vi "configure piezo and pockelscontrol for galvo.vi"() -> (0 "error out":errorcluster, 3 "Array of Piezo and Pockels Task":refnum<k21>[](array[refnum]))   [LabVIEW 2017]
doc: "SciScan 1.2 160622"
uses:
  <vilib>/DAQmx/write.llb/DAQmx Write (Analog 2D DBL NChan NSamp).vi
  <vilib>/DAQmx/write.llb/DAQmx Write (Analog 1D DBL 1Chan NSamp).vi
  GFG/GFGstringGet.vi
  GFG/GFGfpRefGet.vi
  GFG/GFGnumericGet.vi
  GFG/GFGbooleanGet.vi
  <vilib>/DAQmx/create/channels.llb/DAQmx Create Channel (AO-Voltage-Basic).vi
  <vilib>/DAQmx/miscellaneous.llb/DAQmx Fill In Error Info.vi
  <vilib>/DAQmx/configure/trigger.llb/DAQmx Start Trigger (Digital Edge).vi
  GFG/GFG library.lvlib
  <resource>/objmgr/daqmx.rc
panel:
  out "error out 2":errorcluster
  out "pockels cell control":dbl[](graph)
  out "piezo control":dbl[](graph)
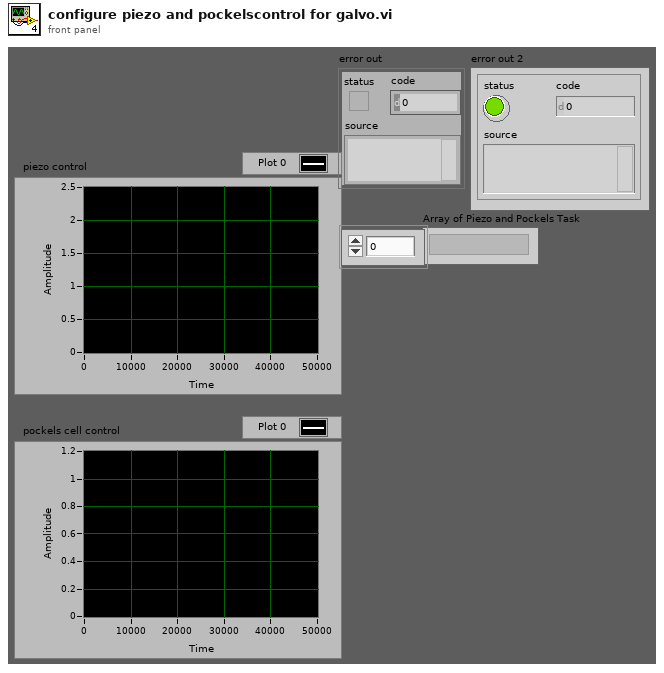
[diagram p1: front panel]
types:
  T1 = enum8{"Enabled", "Disabled", "Disabled and Grayed Out"}
  T2 = cluster{"WaveformChartRef":refnum<vi>, "DigitalRef":refnum<vi>, "ArrayRef":refnum<vi>, "TabControlRef":refnum<vi>, "EnumRef":refnum<vi>, "RingRef":refnum<vi>, "BooleanRef":refnum<vi>, "KnobRef":refnum<vi>, "SlideRef":refnum<vi>, "PathRef":refnum<vi>, "StringRef":refnum<vi>, "ComboBox":refnum<vi>, "WaveformGraphRef":refnum<vi>}
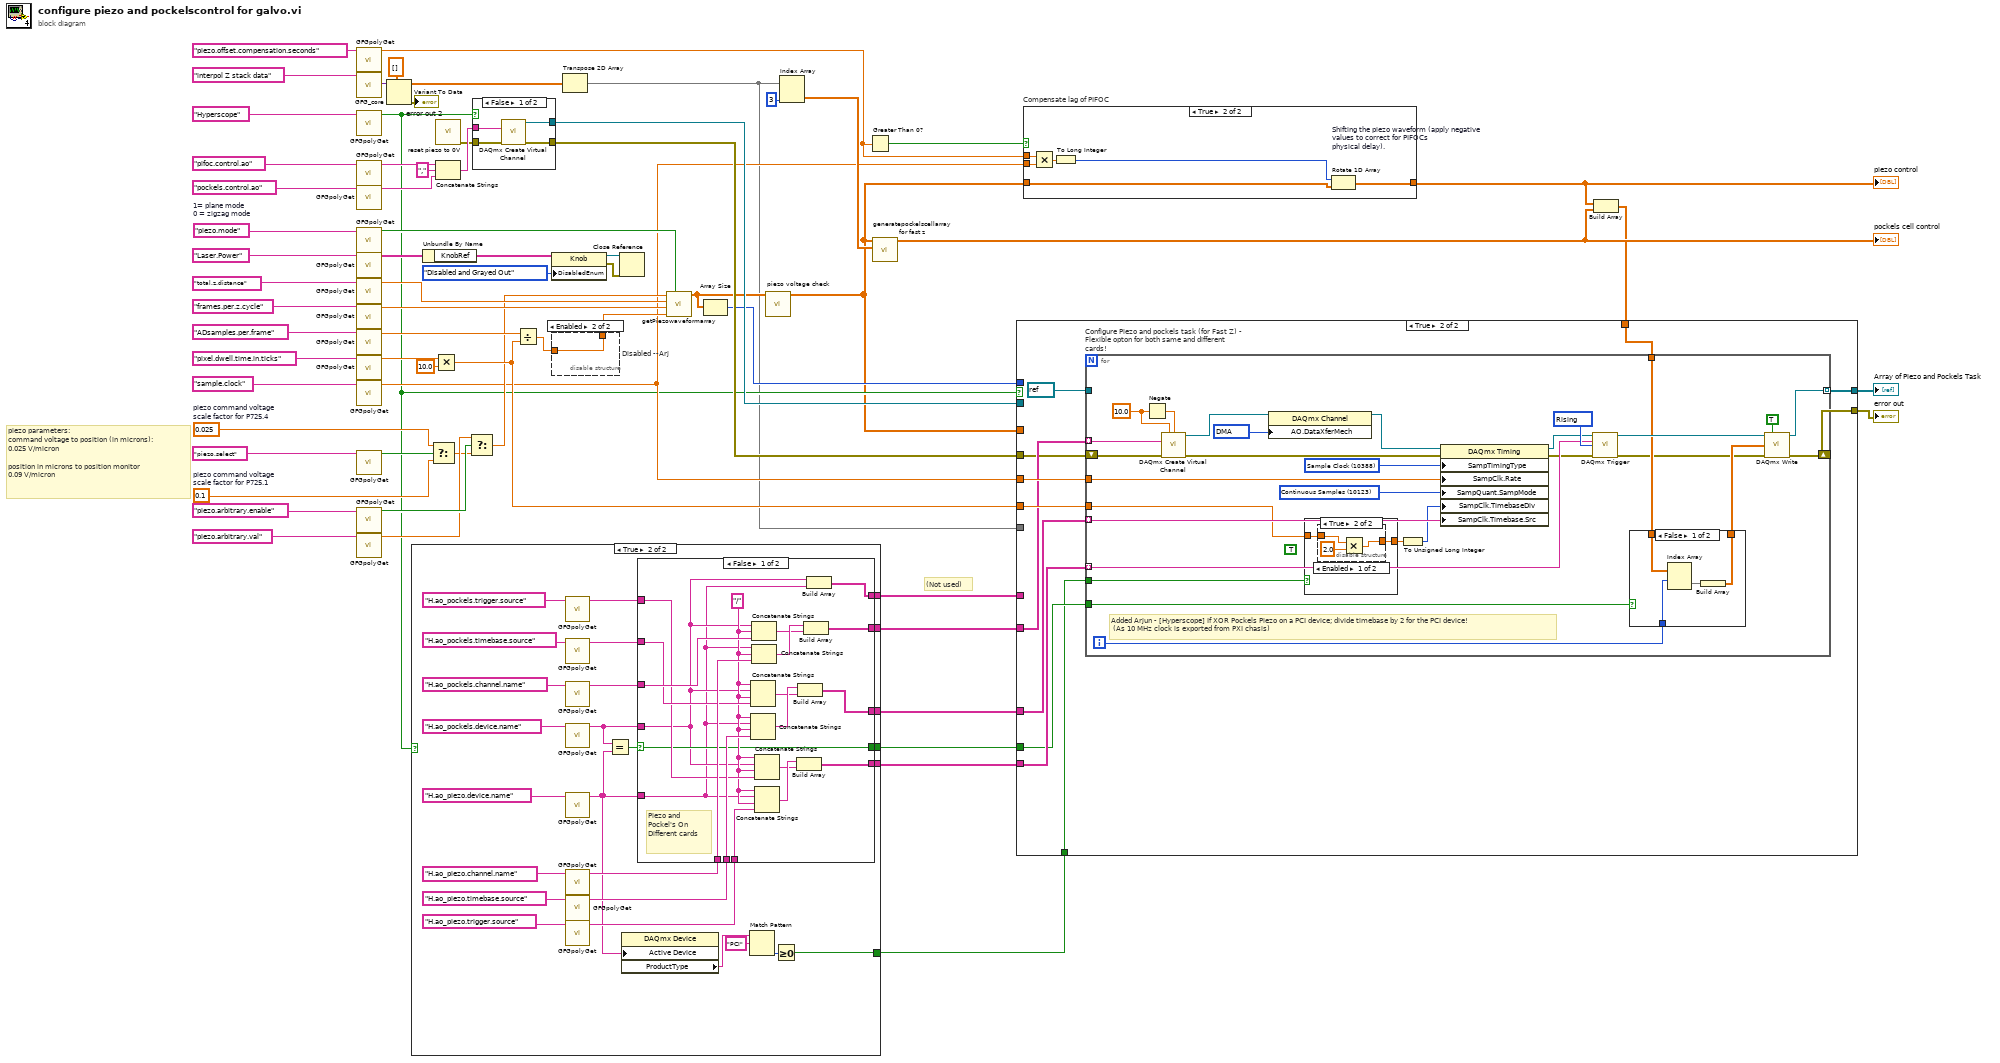
[diagram p0: block diagram]
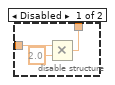
[diagram p2: hidden frame]
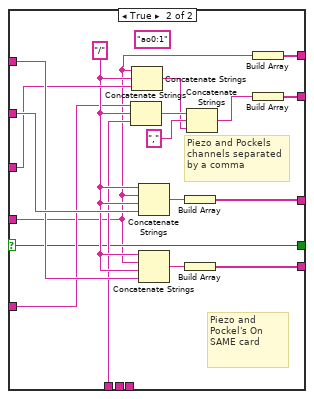
[diagram p4: hidden frame]
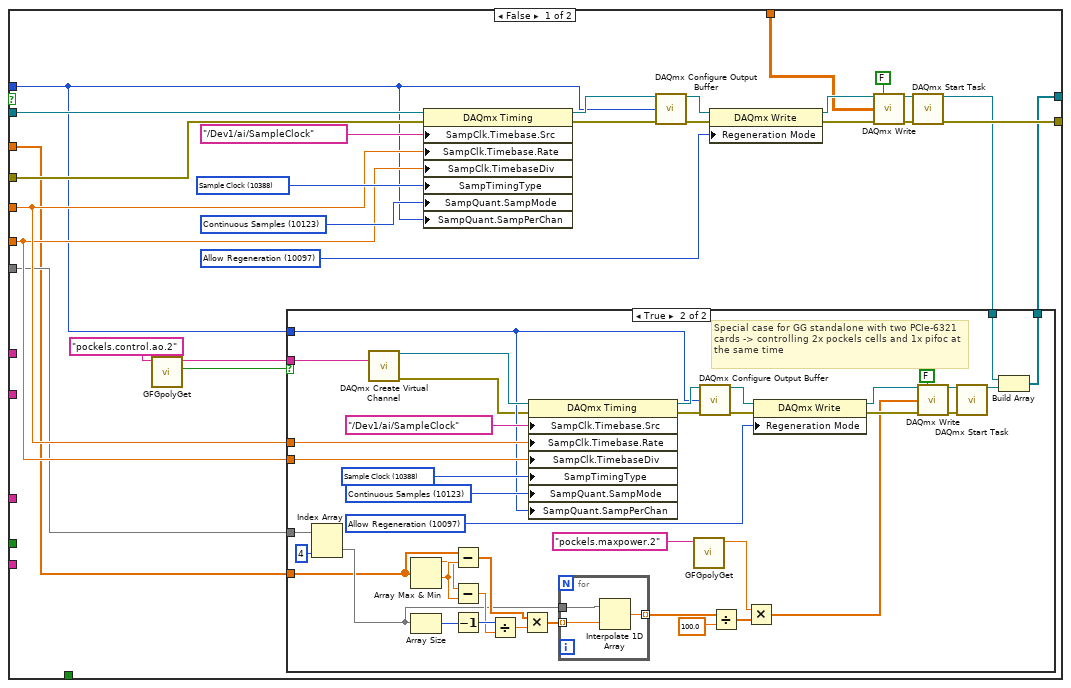
[diagram p6: hidden frame]
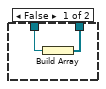
[diagram p7: hidden frame]
diagram:
  w37 = 0.1  # piezo command voltage scale factor for P725.1
  w38 = 0.025  # piezo command voltage scale factor for P725.4
  w48 = "piezo.mode"  # 1= plane mode 0 = zigzag mode
  # "(Not used)"
  # "piezo parameters:\ncommand voltage to position (in microns):\n0.025 V/micron\n\nposition in microns to position monitor\n0.09 V/micron"
  n1 = call-poly "GFGpolyGet.vi"("Variable Name in"="piezo.offset.compensation.seconds") -> ("Numeric"=w16:dbl)  [unwired: 8 in, 2 out]
  n2 = call "GFG_core.vi"("Variable Name in"="interpol Z stack data") -> ("Variant Out"=w47:variant)  [unwired: 12 in, 6 out]
  n3 = call-poly "GFGpolyGet.vi"("Variable Name in"="Hyperscope") -> ("Boolean Value OUT"=w5:bool)  [unwired: 9 in, 1 out]
  n4 = call-poly "GFGpolyGet.vi"("Variable Name in"="pifoc.control.ao") -> ("String"=w65:string)  [unwired: 9 in, 1 out]
  n5 = call-poly "GFGpolyGet.vi"("Variable Name in"="pockels.control.ao" ("Tag in")) -> ("String"=w64:string)  [unwired: 9 in, 1 out]
  n6 = call-poly "GFGpolyGet.vi"("Variable Name in"=w48) -> ("Boolean Value OUT"=w43:bool)  [unwired: 9 in, 1 out]
  n7 = call-poly "GFGpolyGet.vi"("Variable Name in"="Laser.Power") -> ("output cluster"=w62:T2)  [unwired: 9 in, 1 out]
  n8 = call-poly "GFGpolyGet.vi"("Variable Name in"="total.z.distance") -> ("Numeric"=w32:dbl)  [unwired: 8 in, 2 out]
  n9 = call-poly "GFGpolyGet.vi"("Variable Name in"="frames.per.z.cycle" ("Tag in")) -> ("Numeric"=w49:dbl)  [unwired: 8 in, 2 out]
  n10 = call-poly "GFGpolyGet.vi"("Variable Name in"="ADsamples.per.frame" ("Tag in")) -> ("Numeric"=w51:dbl)  [unwired: 8 in, 2 out]
  n11 = call-poly "GFGpolyGet.vi"("Variable Name in"="pixel.dwell.time.in.ticks" ("Tag in")) -> ("Numeric"=w53:dbl)  [unwired: 8 in, 2 out]
  n12 = call-poly "GFGpolyGet.vi"("Variable Name in"="sample.clock" ("Tag in")) -> ("Numeric"=w14:dbl)  [unwired: 8 in, 2 out]
  n13 = call-poly "GFGpolyGet.vi"("Variable Name in"="piezo.select") -> ("Boolean Value OUT"=w35:bool)  [unwired: 9 in, 1 out]
  n14 = call-poly "GFGpolyGet.vi"("Variable Name in"="piezo.arbitrary.enable") -> ("Boolean Value OUT"=w27:bool)  [unwired: 9 in, 1 out]
  n15 = call-poly "GFGpolyGet.vi"("Variable Name in"="piezo.arbitrary.val" ("Tag in")) -> ("Numeric"=w26:dbl)  [unwired: 8 in, 2 out]
  n16 = Variant To Data(type=dbl[][] [] ("Interpolated Data"), Variant=w47) -> (data=w45:dbl[][], error out=→"error out 2":errorcluster)  [unwired: 1 in]
  n17 = case shown="True" w5 {
    tunnel: [_ w79] -> w21
    tunnel: [_ w78] -> w20
    tunnel: [_ w77] -> w19
    tunnel: [_ w75] -> w6
    tunnel: [_ w74] -> w2
    tunnel: [_ w69] -> w1
    frame False {
    }
    frame True {
      n18 = call-poly "GFGpolyGet.vi"("Variable Name in"="H.ao_pockels.trigger.source" ("Tag in")) -> ("String"=w80:string)  [unwired: 9 in, 1 out]
      n19 = call-poly "GFGpolyGet.vi"("Variable Name in"="H.ao_pockels.timebase.source" ("Tag in")) -> ("String"=w81:string)  [unwired: 9 in, 1 out]
      n20 = call-poly "GFGpolyGet.vi"("Variable Name in"="H.ao_pockels.channel.name" ("Tag in")) -> ("String"=w82:string)  [unwired: 9 in, 1 out]
      n21 = call-poly "GFGpolyGet.vi"("Variable Name in"="H.ao_pockels.device.name" ("Tag in")) -> ("String"=w92:string)  [unwired: 9 in, 1 out]
      n22 = call-poly "GFGpolyGet.vi"("Variable Name in"="H.ao_piezo.device.name" ("Tag in")) -> ("String"=w70:string)  [unwired: 9 in, 1 out]
      n23 = call-poly "GFGpolyGet.vi"("Variable Name in"="H.ao_piezo.channel.name" ("Tag in")) -> ("String"=w85:string)  [unwired: 9 in, 1 out]
      n24 = call-poly "GFGpolyGet.vi"("Variable Name in"="H.ao_piezo.timebase.source" ("Tag in")) -> ("String"=w84:string)  [unwired: 9 in, 1 out]
      n25 = call-poly "GFGpolyGet.vi"("Variable Name in"="H.ao_piezo.trigger.source" ("Tag in")) -> ("String"=w83:string)  [unwired: 9 in, 1 out]
      n26 = Equal?(x=w92, y=w70) -> (x = y?=w76:bool)
      n27 = property class="DAQmx Device"("Active Device"=w70) -> ("ProductType"=w73:string)  [unwired: 2 in, 2 out]
      n28 = case shown="False" w76 {
        selector: w76 -> [w98 w117]
        tunnel: w92 -> [w97 w116]
        tunnel: w85 -> [w113 w123]
        tunnel: w84 -> [w110 _]
        tunnel: w83 -> [w107 _]
        tunnel: w70 -> [w96 w122]
        tunnel: w82 -> [w114 w125]
        tunnel: w81 -> [w111 w131]
        tunnel: w80 -> [w109 w126]
        tunnel: [w112 w132] -> w79
        tunnel: [w105 w129] -> w78
        tunnel: [w106 w127] -> w77
        tunnel: [w98 w117] -> w75
        tunnel: [w95 w115] -> w74
        frame False {
          w108 = "/" ("Tag in")
          # "Piezo and Pockel's On Different cards"
          n29 = Concatenate Strings(w108, w97, w108, w111) -> (w101:string)
          n30 = Concatenate Strings(w108, w96, w108, w110) -> (w102:string)
          n31 = Concatenate Strings(w97, w108, w114) -> (w103:string)
          n32 = Concatenate Strings(w96, w108, w113) -> (w104:string)
          n33 = Concatenate Strings(w108, w97, w108, w109) -> (w99:string)
          n34 = Concatenate Strings(w108, w96, w108, w107) -> (w100:string)
          n35 = Build Array(w100, w99) -> (w106:string[])
          n36 = Build Array(w102, w101) -> (w105:string[])
          n37 = Build Array(w104, w103) -> (w112:string[])
          n38 = Build Array(w97, w96) -> (w95:string[])
        }
        frame True {
          (unwired) "ao0:1" ("string")
          w124 = "/" ("Tag in")
          # "Piezo and Pockels channels separated by a comma"
          # "Piezo and Pockel's On SAME card"
          n39 = Concatenate Strings(w122, w124, w123) -> (w121:string)
          n40 = Concatenate Strings(w116, w124, w125) -> (w119:string)
          n41 = Concatenate Strings(w124, w116, w124, w131) -> (w130:string)
          n42 = Concatenate Strings(w124, w116, w124, w126) -> (w128:string)
          n43 = Build Array(w130) -> (w129:string[])
          n44 = Build Array(w128) -> (w127:string[])
          n45 = Concatenate Strings(w121, "," ("string"), w119) -> (w118:string)
          n46 = Build Array(w116) -> (w115:string[])
          n47 = Build Array(w118) -> (w132:string[])
        }
      }
      n48 = Match Pattern(string=w73, regular expression="PCI") -> (offset past match=w71:i32)  [unwired: 1 in, 3 out]
      n49 = Greater Or Equal To 0?(x=w71) -> (x >= 0?=w69:bool)
    }
  }
  n50 = Unbundle By Name(w62) -> ("KnobRef"=w61:refnum<vi>)
  n51 = Select(t=w38, s=w35, f=w37) -> (s? t:f=w25:dbl)
  n52 = Multiply(x=w53, y=10.0) -> (x*y=w31:dbl)
  n53 = call "reset piezo to 0V.vi"() -> ("error out"=w40:errorcluster)  [unwired: 11 in]
  n54 = Concatenate Strings(w65, "," ("string"), w64) -> (w55:string)
  n55 = Select(t=w26, s=w27, f=w25) -> (s? t:f=w24:dbl)
  n56 = case shown="False" w5 {
    tunnel: [w136 w137] -> w59
    tunnel: [w135 _] -> w58
    tunnel: w55 -> [w134 _]
    tunnel: w40 -> [w133 w137]
    frame False {
      n57 = call-poly <vilib>:"DAQmx Create Virtual Channel.vi"("physical channels"=w134, "error in"=w133) -> ("task out"=w135:refnum<k21>, "error out"=w136:errorcluster)  [unwired: 12 in]
    }
    frame True {
    }
  }
  n58 = Divide(x=w51, y=w31) -> (x/y=w7:dbl)
  n59 = property class="Knob"(reference=w61, "DisabledEnum"=T1."Disabled and Grayed Out" ("Disabled")) -> (reference out=w9:refnum<vi>, error out=w8:errorcluster)  [unwired: 1 in]
  n60 = disable-structure "Disabled --Arj" shown="Enabled" {
    disable-tunnel: [w140 w141] -> w57
    disable-tunnel: w7 -> [w139 w141]
    frame Disabled {
      n61 = Multiply(x=w139, y=2.0) -> (x*y=w140:dbl)
    }
    frame Enabled {
    }
  }
  n62 = Transpose 2D Array(2D array=w45) -> (transposed array=w4:dbl[][])
  n63 = Close Reference(reference=w9, error in (no error)=w8) -> ()  [unwired: 1 out]
  n64 = call "getPiezowaveformarray.vi"("sawtooth or zigzag"=w43, "pixel.num"=w57, "frames.per.z.cycle"=w49, "total.z.distance"=w32, "piezo scale factor"=w24) -> ("Array"=w13:dbl[])  [unwired: 6 in]
  n65 = Array Size(array=w13) -> (size(s)=w56:i32)
  n66 = call "piezo voltage check.vi"("piezo array in"=w13) -> ("piezo array out"=w3:dbl[])  [unwired: 10 in]
  n67 = Index Array(array=w4, index (col)=3 ("disabled index (col)")) -> (element=w42:dbl[])  [unwired: 1 in]
  n68 = Greater Than 0?(x=w16) -> (x > 0?=w15:bool)
  n69 = call "generatepockelscellarray for fast z.vi"("interpolated pockels cell data"=w42, "piezo control"=w3) -> ("pockelscellarray"=w11:dbl[])  [unwired: 9 in]
  "pockels cell control" <- w11
  n70 = case "Compensate lag of PIFOC" shown="True" w15 {
    tunnel: w3 -> [w142 w145]
    tunnel: [w142 w143] -> w12
    tunnel: w16 -> [_ w148]
    tunnel: w14 -> [_ w146]
    frame False {
    }
    frame True {
      n71 = Multiply(x=w148, y=w146) -> (x*y=w147:dbl)
      n72 = To Long Integer(number=w147) -> (32bit integer=w144:i32)
      n73 = Rotate 1D Array "Shifting the piezo waveform (apply negative values to correct for PIFOCs\nphysical delay)."(1:w145, 2:w144) -> (0:w143:dbl[])
    }
  }
  "piezo control" <- w12
  n74 = Build Array(w12, w11) -> (w10:dbl[][])
  n75 = case shown="True" w5 {
    tunnel: w59 -> [w169 w224]
    tunnel: w58 -> [w167 _]
    tunnel: w56 -> [w151 _]
    tunnel: w10 -> [w156 w232]
    tunnel: w14 -> [w153 w230]
    tunnel: [w154 w231] -> w18
    tunnel: [w160 w223] -> w39
    tunnel: w31 -> [w152 w229]
    tunnel: w21 -> [_ w226]
    tunnel: w20 -> [_ w227]
    tunnel: w19 -> [_ w228]
    tunnel: w6 -> [_ w225]
    tunnel: w4 -> [w150 _]
    tunnel: w3 -> [w149 _]
    tunnel: w2 -> [_ _]
    tunnel: w1 -> [_ w221]
    frame False {
      w166 = 10388 items=["Sample Clock"=10388, "Burst Handshake"=12548, "Handshake"=10389, "Implicit"=10451, "On Demand"=10390, "Change Detection"=12504, "Pipelined Sample Clock"=14668] ("SampTimingType")
      w174 = 10097 items=["Allow Regeneration"=10097, "Do Not Allow Regeneration"=10158] ("RegenMode")
      w165 = 10123 items=["Finite Samples"=10178, "Continuous Samples"=10123] ("sample mode")
      n76 = call-poly "GFGpolyGet.vi"("Variable Name in"="pockels.control.ao.2" ("Tag in")) -> ("Found/Replaced"=w158:bool, "String"=w157:string)  [unwired: 9 in]
      n77 = property class="DAQmx Timing"(reference=w167, error in=w169, "SampClk.Timebase.Src"=tag "/Dev1/ai/SampleClock" ("Clock Source"), "SampClk.Timebase.Rate"=w153, "SampClk.TimebaseDiv"=w152, "SampTimingType"=w166, "SampQuant.SampMode"=w165, "SampQuant.SampPerChan"=w151) -> (reference out=w163:refnum<k21>, error out=w170:errorcluster)
      n78 = call <vilib>:"DAQmx Configure Output Buffer.vi"("task/channels in"=w163, "buffer size (in samples per channel)"=w151, "error in"=w170) -> ("task out"=w175:refnum<k21>, "error out"=w173:errorcluster)  [unwired: 11 in]
      n79 = property class="DAQmx Write"(reference=w175, error in=w173, "Regeneration Mode"=w174) -> (reference out=w171:refnum<k21>, error out=w172:errorcluster)
      n80 = call-poly <vilib>:"DAQmx Write.vi"("task/channels in"=w171, "auto start"=FALSE, "data"=w156, "error in"=w172) -> ("task out"=w162:refnum<k21>, "error out"=w164:errorcluster)  [unwired: 9 in, 1 out]
      n81 = call <vilib>:"DAQmx Start Task.vi"("task/channels in"=w162, "error in"=w164) -> ("task out"=w155:refnum<k21>, "error out"=w160:errorcluster)  [unwired: 12 in]
      n82 = case shown="True" w158 {
        tunnel: w157 -> [_ w217]
        tunnel: w155 -> [w177 w202]
        tunnel: [w176 w200] -> w154
        tunnel: w153 -> [_ w199]
        tunnel: w152 -> [_ w198]
        tunnel: w151 -> [_ w197]
        tunnel: w150 -> [_ w194]
        tunnel: w149 -> [_ w178]
        frame False {
          n83 = Build Array(w177) -> (w176:refnum<k21>[])
        }
        frame True {
          w211 = 10388 items=["Sample Clock"=10388, "Burst Handshake"=12548, "Handshake"=10389, "Implicit"=10451, "On Demand"=10390, "Change Detection"=12504, "Pipelined Sample Clock"=14668] ("SampTimingType")
          w205 = 10097 items=["Allow Regeneration"=10097, "Do Not Allow Regeneration"=10158] ("RegenMode")
          w212 = 10123 items=["Finite Samples"=10178, "Continuous Samples"=10123] ("sample mode")
          # "Special case for GG standalone with two PCIe-6321 cards -> controlling 2x pockels cells and 1x pifoc at the same time"
          n84 = Index Array(array=w194, index (col)=4 ("disabled index (col)")) -> (element=w180:dbl[])  [unwired: 1 in]
          n85 = call-poly <vilib>:"DAQmx Create Virtual Channel.vi"("physical channels"=w217) -> ("task out"=w203:refnum<k21>, "error out"=w196:errorcluster)  [unwired: 13 in]
          n86 = Array Max & Min(array=w178) -> (max value=w183:dbl, min value=w186:dbl)  [unwired: 2 out]
          n87 = Array Size(array=w180) -> (size(s)=w181:i32)
          n88 = Subtract(x=w178, y=w186) -> (x-y=w185:dbl[])
          n89 = Subtract(x=w183, y=w186) -> (x-y=w184:dbl)
          n90 = Decrement(x=w181) -> (x-1=w193:i32)
          n91 = Divide(x=w193, y=w184) -> (x/y=w182:dbl)
          n92 = Multiply(x=w185, y=w182) -> (x*y=w187:dbl[])
          n93 = property class="DAQmx Timing"(reference=w203, error in=w196, "SampClk.Timebase.Src"=tag "/Dev1/ai/SampleClock" ("Clock Source"), "SampClk.Timebase.Rate"=w199, "SampClk.TimebaseDiv"=w198, "SampTimingType"=w211, "SampQuant.SampMode"=w212, "SampQuant.SampPerChan"=w197) -> (reference out=w214:refnum<k21>, error out=w209:errorcluster)
          n94 = for {
            tunnel: w180 -> [w220]
            tunnel: [w219] -> w190 mode=indexing
            tunnel: w187 -> [w218] mode=indexing
            n95 = Interpolate 1D Array(1:w218, 2:w220) -> (0:w219:dbl)
          }
          n96 = call-poly "GFGpolyGet.vi"("Variable Name in"="pockels.maxpower.2") -> ("Numeric"=w192:dbl)  [unwired: 8 in, 2 out]
          n97 = call <vilib>:"DAQmx Configure Output Buffer.vi"("task/channels in"=w214, "buffer size (in samples per channel)"=w197, "error in"=w209) -> ("task out"=w204:refnum<k21>, "error out"=w206:errorcluster)  [unwired: 11 in]
          n98 = Divide(x=w190, y=100.0 ("x")) -> (x/y=w189:dbl[])
          n99 = Multiply(x=w192, y=w189) -> (x*y=w179:dbl[])
          n100 = property class="DAQmx Write"(reference=w204, error in=w206, "Regeneration Mode"=w205) -> (reference out=w208:refnum<k21>, error out=w207:errorcluster)
          n101 = call-poly <vilib>:"DAQmx Write.vi"("task/channels in"=w208, "auto start"=FALSE, "data"=w179, "error in"=w207) -> ("task out"=w215:refnum<k21>, "error out"=w213:errorcluster)  [unwired: 9 in, 1 out]
          n102 = call <vilib>:"DAQmx Start Task.vi"("task/channels in"=w215, "error in"=w213) -> ("task out"=w201:refnum<k21>)  [unwired: 12 in, 1 out]
          n103 = Build Array(w202, w201) -> (w200:refnum<k21>[])
        }
      }
    }
    frame True {
      n104 = for "Configure Piezo and pockels task (for Fast Z) - Flexible opton for both same and different cards!" {
        tunnel: w226 -> [w251] mode=indexing
        tunnel: w232 -> [w246]
        tunnel: w230 -> [w250]
        tunnel: w229 -> [w237]
        tunnel: w228 -> [w248] mode=indexing
        tunnel: w227 -> [w247] mode=indexing
        tunnel: w225 -> [w234]
        shift-right: [w239] -> w223
        shift-left: w224 -> [w243]
        tunnel: refnum<k21> refnum ("task out") -> [_]
        tunnel: [w249] -> w231 mode=indexing
        tunnel: w221 -> [w233]
        i -> [w244]
        (unwired) TRUE
        w238 = 10054 items=["DMA"=10054, "Interrupts"=10204, "Programmed I/O"=10264, "USB Bulk"=12590] ("AO.DataXferMech")
        w252 = 10388 items=["Sample Clock"=10388, "Burst Handshake"=12548, "Handshake"=10389, "Implicit"=10451, "On Demand"=10390, "Change Detection"=12504, "Pipelined Sample Clock"=14668] ("SampTimingType")
        w254 = 10280 items=["Rising"=10280, "Falling"=10171] ("edge")
        w256 = 10123 items=["Finite Samples"=10178, "Continuous Samples"=10123, "Hardware Timed Single Point"=12522] ("SampQuant.SampMode")
        w260 = 10.0 ("maximum value")
        # "Added Arjun - [Hyperscope] If XOR Pockels Piezo on a PCI device; divide timebase by 2 for the PCI device!\n (As 10 MHz clock is exported from PXI chasis)"
        n105 = Negate(x=w260) -> (-x=w261:dbl)
        n106 = call-poly <vilib>:"DAQmx Create Virtual Channel.vi"("maximum value"=w260, "minimum value"=w261, "physical channels"=w251, "error in"=w243) -> ("task out"=w258:refnum<k21>, "error out"=w242:errorcluster)  [unwired: 10 in]
        n107 = property class="DAQmx Channel"(reference=w258, "AO.DataXferMech"=w238) -> (reference out=w255:refnum<k21>)  [unwired: 1 in, 1 out]
        n108 = case shown="True" w233 {
          tunnel: w237 -> [w262 w264]
          tunnel: [w262 w263] -> w236
          frame False {
          }
          frame True {
            n109 = disable-structure shown="Enabled" {
              disable-tunnel: w264 -> [w267 w268]
              disable-tunnel: [w265 w268] -> w263
              frame Enabled {
                n110 = Multiply(x=w267, y=2.0) -> (x*y=w265:dbl)
              }
              frame Disabled {
              }
            }
          }
        }
        n111 = To Unsigned Long Integer(number=w236) -> (unsigned 32bit integer=w235:u32)
        n112 = property class="DAQmx Timing"(reference=w255, error in=w242, "SampTimingType"=w252, "SampClk.Rate"=w250, "SampQuant.SampMode"=w256, "SampClk.TimebaseDiv"=w235, "SampClk.Timebase.Src"=w247) -> (reference out=w253:refnum<k21>, error out=w241:errorcluster)
        n113 = call-poly <vilib>:"DAQmx Trigger.vi"("task/channels in"=w253, "source"=w248, "edge"=w254, "error in"=w241) -> ("task out"=w257:refnum<k21>, "error out"=w240:errorcluster)  [unwired: 10 in]
        n114 = case shown="False" w234 {
          tunnel: w246 -> [w272 w273]
          tunnel: [w269 w273] -> w245
          tunnel: w244 -> [w271 _]
          frame False {
            n115 = Index Array(array=w272, index (row)=w271) -> (element=w270:dbl[])  [unwired: 1 in]
            n116 = Build Array(w270) -> (w269:dbl[][])
          }
          frame True {
          }
        }
        n117 = call-poly <vilib>:"DAQmx Write.vi"("task/channels in"=w257, "auto start"=TRUE, "data"=w245, "error in"=w240) -> ("task out"=w249:refnum<k21>, "error out"=w239:errorcluster)  [unwired: 9 in, 1 out]
      }
    }
  }
  "error out" <- w39
  "Array of Piezo and Pockels Task" <- w18
